vi "Occurrences.vi"() -> ()   [LabVIEW 2012]
panel:
  out "LED 2":bool
  out "LED":bool
  in  "Set Occurrence":bool
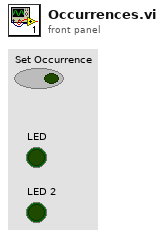
[diagram p1: front panel]
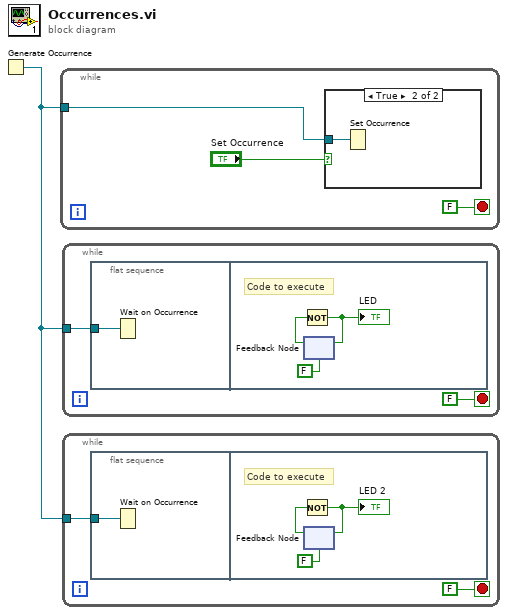
[diagram p0: block diagram]
diagram:
  n1 = Generate Occurrence() -> (w1:refnum<k4>)
  n2 = while {
    tunnel: w1 -> [w4]
    stop <- FALSE stop-if-true
    n3 = case shown="True" "Set Occurrence" {
      tunnel: w4 -> [_ w5]
      frame False {
      }
      frame True {
        n4 = Set Occurrence(w5) -> ()
      }
    }
  }
  n5 = while {
    tunnel: w1 -> [w7]
    stop <- FALSE stop-if-true
    n6 = flat-sequence {
      tunnel: w7 -> [w8]
      frame #0 {
        n7 = Wait on Occurrence(2:w8) -> ()  [unwired: 2 in, 1 out]
      }
      frame #1 {
        # "Code to execute"
        n8 = feedback #1(FALSE) -> (w11:bool)
        n9 = Not(x=w11) -> (.not. x?=w10:bool)
        "LED" <- w10
        n10 = feedback-in #1(w10) -> ()
      }
    }
  }
  n11 = while {
    tunnel: w1 -> [w13]
    stop <- FALSE stop-if-true
    n12 = flat-sequence {
      tunnel: w13 -> [w14]
      frame #0 {
        n13 = Wait on Occurrence(2:w14) -> ()  [unwired: 2 in, 1 out]
      }
      frame #1 {
        # "Code to execute"
        n14 = feedback #2(FALSE) -> (w17:bool)
        n15 = Not(x=w17) -> (.not. x?=w16:bool)
        "LED 2" <- w16
        n16 = feedback-in #2(w16) -> ()
      }
    }
  }
